vi "Bitfile Component Check.vi"(1 "Control Scalars":T1) -> (0 "Valid?":bool)   [LabVIEW 2011, in "Engine Sim System Explorer.lvlib"]
uses:
  <userlib>/_FPGA Interface Advanced Tools/FPGA Bitfile Utility/TypeDefs/Scalar Register Set.ctl
  <userlib>/_FPGA Interface Advanced Tools/FPGA Bitfile Utility/TypeDefs/Scalar Register.ctl
  Engine Sim System Explorer.lvlib
  <userlib>/_FPGA Interface Advanced Tools/FPGA Bitfile Utility/FPGA Bitfile Utility.lvlib
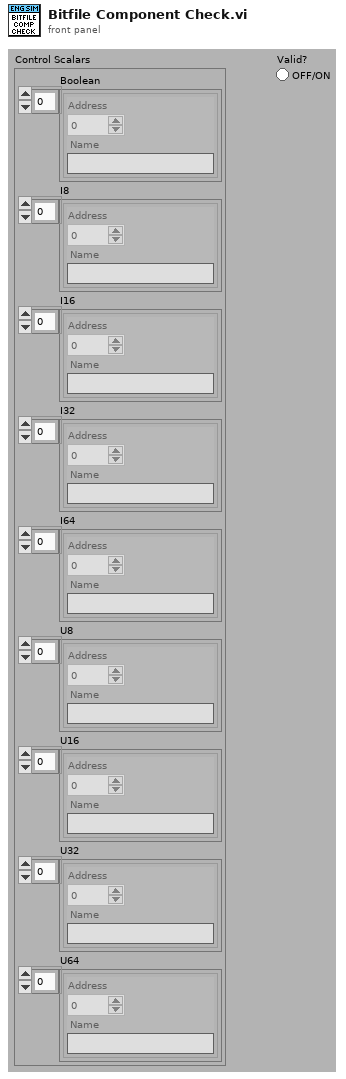
[diagram p1: front panel]
types:
  T1 = typedef "FPGA Bitfile Utility.lvlib/Scalar Register Set.ctl" = cluster{"Boolean":T2[], "I8":T2[], "I16":T2[], "I32":T2[], "I64":T2[], "U8":T2[], "U16":T2[], "U32":T2[], "U64":T2[]}
  T2 = typedef "FPGA Bitfile Utility.lvlib/Scalar Register.ctl" = cluster{"Address":u32, "Name":string}
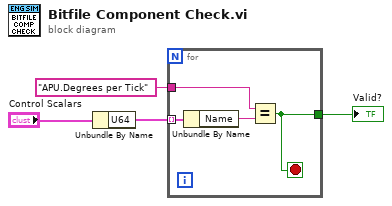
[diagram p0: block diagram]
diagram:
  n1 = Unbundle By Name("Control Scalars") -> ("U64"=w3:T2[])
  n2 = for {
    tunnel: w3 -> [w8] mode=indexing
    tunnel: "APU.Degrees per Tick" ("Item Path in") -> [w6]
    tunnel: [w5] -> w1
    stop <- w5 stop-if-true
    n3 = Unbundle By Name(w8) -> ("Name"=w7:string)
    n4 = Equal?(x=w6, y=w7) -> (x = y?=w5:bool)
  }
  "Valid?" <- w1
